vi "Build GPIO Waveform.vi"(0 "gpio timestamps in":T3(array[cluster]), 5 "gpio to display":T1[](array[typedef]), 9 "min timestamp id":T2=enum."Ser0 GPIO Bank") -> (4 "parsing error":bool, 6 "waveform out":digitalwaveform[](array[waveform]))   [LabVIEW 2023, in "GettingStarted_Common_148X_Host.lvlib"]
uses:
  GettingStarted_Common_148X_Host.lvlib
  <instrlib>/FlexRIO/CSI-2/v2/FPGA/Types/Timestamp ID.ctl
  Types/GPIO Filter.ctl
  <vilib>/Waveform/DWDTOps.llb/DWDT Append Digital Signals.vi
  <vilib>/Waveform/DWDTOps.llb/DWDT Digital Signal Subset.vi
  <vilib>/regexp/Match Regular Expression.xnode
  <instrlib>/FlexRIO/CSI-2/v2/FPGA/NI CSI-2 API FPGA v2.lvlib
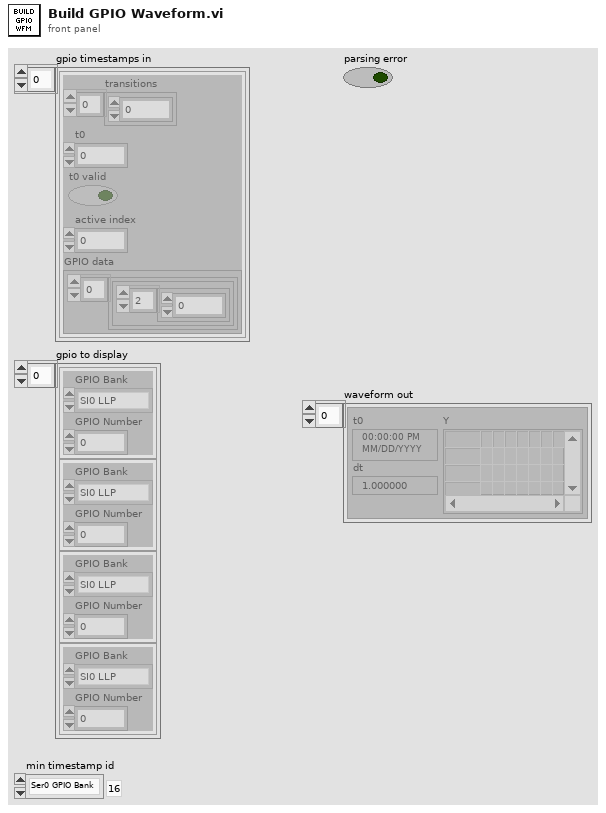
[diagram p1: front panel]
types:
  T1 = typedef "GettingStarted_Common_148X_Host.lvlib/GPIO Filter.ctl" = cluster{"GPIO Bank":T2, "GPIO Number":i32}
  T2 = typedef "NI CSI-2 API FPGA v2.lvlib/Timestamp ID.ctl" = enum8{"SI0 LLP", "SI1 LLP", "SI2 LLP", "SI3 LLP", "SI4 LLP", "SI5 LLP", "SI6 LLP", "SI7 LLP", "SO0 LLP", "SO1 LLP", "SO2 LLP", "SO3 LLP", "SO4 LLP", "SO5 LLP", "SO6 LLP", "SO7 LLP", "Ser0 GPIO Bank", "Ser1 GPIO Bank", "Ser2 GPIO Bank", "Ser3 GPIO Bank", "Ser4 GPIO Bank", "Ser5 GPIO Bank", "Ser6 GPIO Bank", "Ser7 GPIO Bank", "Des0 GPIO Bank", "Des1 GPIO Bank", "Des2 GPIO Bank", "Des3 GPIO Bank", "Des4 GPIO Bank", "Des5 GPIO Bank", "Des6 GPIO Bank", "Des7 GPIO Bank", "User0", "User1", "User2", "User3", "User4", "User5", "User6", "User7", "User8", "User9", "User10", "User11", "User12", "User13", "User14", "User15", "User16", "User17", "User18", "User19", "User20", "User21", "User22", "User23", "User24", "User25", "User26", "User27", "User28", "User29", "User30", "User31"}
  T3 = cluster{"transitions":u64[], "t0":u64, "t0 valid":bool, "active index":i32, "GPIO data":cluster{cluster{u8[]}[]}}[]
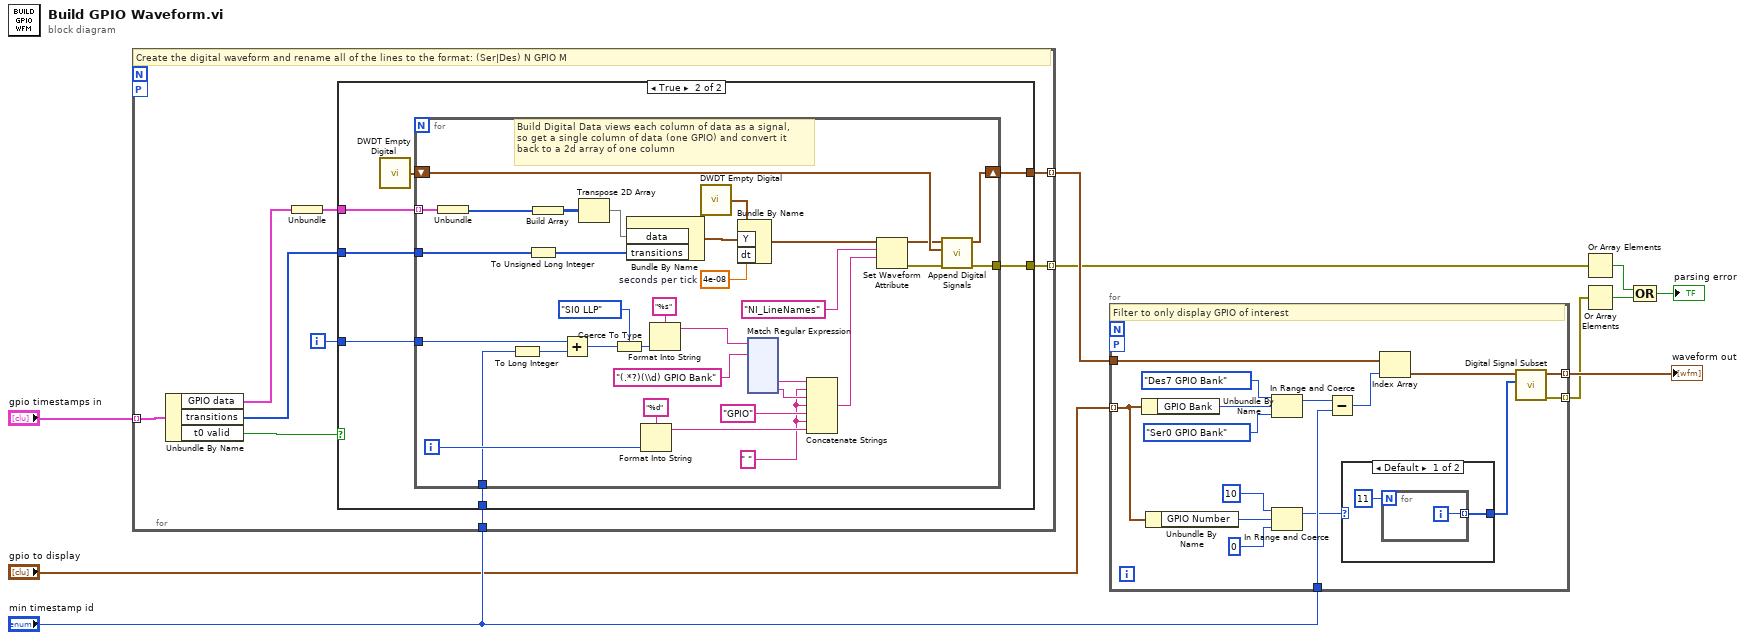
[diagram p0: block diagram]
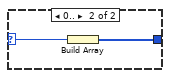
[diagram p3: hidden frame]
diagram:
  n1 = for {
    tunnel: [w19] -> w2 mode=indexing
    tunnel: [w18] -> w9 mode=indexing
    tunnel: "gpio timestamps in" -> [w16] mode=indexing
    tunnel: "min timestamp id" -> [w13]
    workers-P: _ -> [_]
    i -> [w17]
    # "Create the digital waveform and rename all of the lines to the format: (Ser|Des) N GPIO M"
    n2 = Unbundle By Name(w16) -> ("GPIO data"=w12:cluster{cluster{u8[]}[]}, "transitions"=w15:u64[], "t0 valid"=w11:bool)
    n3 = Unbundle(w12) -> (w14:cluster{u8[]}[])
    n4 = case shown="True" w11 {
      tunnel: [_ w26] -> w19
      tunnel: [_ w20] -> w18
      tunnel: w17 -> [_ w25]
      tunnel: w15 -> [_ w24]
      tunnel: w14 -> [_ w23]
      tunnel: w13 -> [_ w22]
      frame False {
        # "No timestamps collected on this GPIO Bank"
      }
      frame True {
        n5 = call <vilib>:"DWDT Empty Digital.vi"() -> ("digital waveform out"=w21:digitalwaveform)  [unwired: 5 in]
        n6 = for {
          tunnel: [w38] -> w26
          shift-right: [w30] -> w20
          shift-left: w21 -> [w55]
          tunnel: w25 -> [w41]
          tunnel: w22 -> [w37]
          tunnel: w24 -> [w36]
          tunnel: w23 -> [w34] mode=indexing
          i -> [w40]
          w29 = 4e-08  # seconds per tick
          w43 = " " ("string")
          # "Build Digital Data views each column of data as a signal,\nso get a single column of data (one GPIO) and convert it\nback to a 2d array of one column"
          n7 = Unbundle(w34) -> (w35:u8[])
          n8 = To Long Integer(number=w37) -> (32bit integer=w28:i32)
          n9 = To Unsigned Long Integer(number=w36) -> (unsigned 32bit integer=w27:u32[])
          n10 = Build Array(w35) -> (w33:u8[][])
          n11 = Add(x=w41, y=w28) -> (x+y=w50:i32)
          n12 = Transpose 2D Array(2D array=w33) -> (transposed array=w32:u8[][])
          n13 = Coerce To Type(0:w50, 1:Timestamp_ID."SI0 LLP" ("id")) -> (2:w53:T2)
          n14 = Bundle By Name("data"=w32, "transitions"=w27) -> (w59:digitaldata)  [unwired: 1 in]
          n15 = Format Into String(format string="%d", w40) -> (resulting string=w44:string)  [unwired: 2 in, 1 out]
          n16 = Format Into String(format string="%s", w53) -> (resulting string=w51:string)  [unwired: 2 in, 1 out]
          n17 = call <vilib>:"DWDT Empty Digital.vi"() -> ("digital waveform out"=w56:digitalwaveform)  [unwired: 5 in]
          n18 = Bundle By Name(cluster=w56, "Y"=w59, "dt"=w29) -> (w58:digitalwaveform)
          n19 = xnode "Match Regular Expression"("input string"=w51, "regular expression"="(.*?)(\\d) GPIO Bank") -> ("submatch 1"=w48:string, "submatch 2"=w47:string)  [unwired: 4 in, 5 out]
          n20 = Concatenate Strings(w48, w43, w47, w43, "GPIO" ("string"), w43, w44) -> (w42:string)
          n21 = Set Waveform Attribute(5:w42, 6:"NI_LineNames" ("name"), 7:w58) -> (0:w39:errorcluster, 3:w31:digitalwaveform)  [unwired: 1 in, 1 out]
          n22 = call-poly <vilib>:"Append Digital Signals.vi"("error in (no error)"=w39, "digital waveform (low bits)"=w55, "digital waveform (high bits)"=w31) -> ("error out"=w38:errorcluster, "digital waveform out"=w30:digitalwaveform)  [unwired: 7 in]
        }
      }
    }
  }
  n23 = for {
    tunnel: w9 -> [w195]
    tunnel: [w180] -> w4 mode=indexing
    tunnel: "gpio to display" -> [w190] mode=indexing
    tunnel: [w187] -> w1 mode=indexing
    tunnel: "min timestamp id" -> [w186]
    workers-P: _ -> [_]
    # "Filter to only display GPIO of interest"
    n24 = Unbundle By Name(w190) -> ("GPIO Bank"=w191:T2)
    n25 = Unbundle By Name(w190) -> ("GPIO Number"=w184:i32)
    n26 = In Range and Coerce(upper limit=Timestamp_ID."Des7 GPIO Bank" ("y"), x=w191, lower limit=Timestamp_ID."Ser0 GPIO Bank" ("y")) -> (coerced(x)=w194:T2)  [unwired: 1 out]
    n27 = In Range and Coerce(upper limit=10, x=w184, lower limit=0 ("upper limit")) -> (coerced(x)=w183:i32)  [unwired: 1 out]
    n28 = Subtract(x=w194, y=w186) -> (x-y=w188:u8)
    n29 = case shown="Default" w183 {
      selector: w183 -> [_ w199]
      tunnel: [w196 w200] -> w189
      frame Default {
        n30 = for {
          N: 11 -> [_]
          tunnel: [w198] -> w196 mode=indexing
          i -> [w198]
        }
      }
      frame 0.. {
        n31 = Build Array(w199) -> (w200:i32[])
      }
    }
    n32 = Index Array(array=w195, index=w188) -> (element=w185:digitalwaveform)
    n33 = call-poly <vilib>:"Digital Signal Subset.vi"("signals"=w189, "digital waveform"=w185) -> ("error out"=w187:errorcluster, "digital subset"=w180:digitalwaveform)  [unwired: 8 in]
  }
  "waveform out" <- w4
  n34 = Or Array Elements(Boolean array=w2) -> (logical OR=w6:bool)
  n35 = Or Array Elements(Boolean array=w1) -> (logical OR=w7:bool)
  n36 = Compound Arithmetic op=OR(w6, w7) -> (→"parsing error":bool)
